vi "Power Meter Control Panel (No Objects).vi"(8 "error in (no error)":errorcluster) -> (0 "error out":errorcluster)   [LabVIEW 2012]
doc: "(Dynamic) A user-level application that simulates the physical front panel of the Instrument. Provide the user with buttons to manually control features of the instrument, and provide indicators of its current state."
uses:
  Newport 1830-C/Public/Filters.ctl
panel:
  in  "Which Filter":T1=1 items=["Orange"=1, "Green"=2, "Yellow"=3]
  out "Actual Power":dbl
  in  "Measured Power":dbl
  in  "Convert Power":bool
  in  "VISA Resource Name":refnum<visa-resource-name>="GPIB0::4::INSTR"
  out "Initialized?":bool
  in  "Filter":T1=1 items=["Orange"=1, "Green"=2, "Yellow"=3]
  out "Power":string
  in  "Time between Reads (ms)":i32=200
  in  "Read Continuous":bool
  in  "Averaging Time (s)":dbl=0.5
  in  "Averaging":bool
  out "Units":u16(ring)=1 items=["W"=1, "dB"=2, "dBm"=3, "REL"=4]
  out "AVG":u16(ring)=2 items=["Slow"=1, "Medium"=2, "Fast"=3]
  out "Run/Stop":u16(ring) items=["Stop", "Run"]
  out "ATTN":u16(ring) items=["Off", "On"]
  out "Local Lockout":u16(ring) items=["Off", "On"]
  out "Zero":u16(ring) items=["Off", "On"]
  out "Beeper":u16(ring) items=["Off", "On"]
  out "Backlight":u16(ring) items=["Off", "Low", "High"]
  out "Range":u16(ring) items=["Auto", "Highest Sensitivity", "30uW", "300uW", "3mW", "30mW", "300mW", "3W", "Lowest Sensitivity"]
  in  "Run/Stop set":u32(ring)=1 items=["Stop", "Run"]
  in  "ATTN set":u32(ring) items=["Off", "On"]
  in  "BKLT set":u32(ring)=1 items=["Off", "Low", "High"]
  in  "Range set":u32(ring) items=["Auto", "Highest Sensitivity", "30uW", "300uW", "3mW", "30mW", "300mW", "3W", "Lowest Sensitivity"]
  in  "Beeper set":u32(ring) items=["Off", "On"]
  in  "AVG set":u32(ring)=2 items=["Slow"=1, "Medium"=2, "Fast"=3]
  in  "Units set":u32(ring)=1 items=["W"=1, "dB"=2, "mdB"=3, "REL"=4]
  in  "Zero set":u32(ring) items=["Off", "On"]
  in  "Local set":u32(ring) items=["Off", "On"]
  in  "Read Current Power":bool
  in  "Set":bool
  in  "Read to \nControl":bool
  in  "Read":bool
  in  "Wavelength Set":dbl[unit]
  out "Wavelength":dbl[unit]
  in  "Copy actual to set":bool
  in  "Populate fields with member data":bool
  in  "stop":bool
  # "With \nAttn\nOn"
  # "Convert Measured Power"
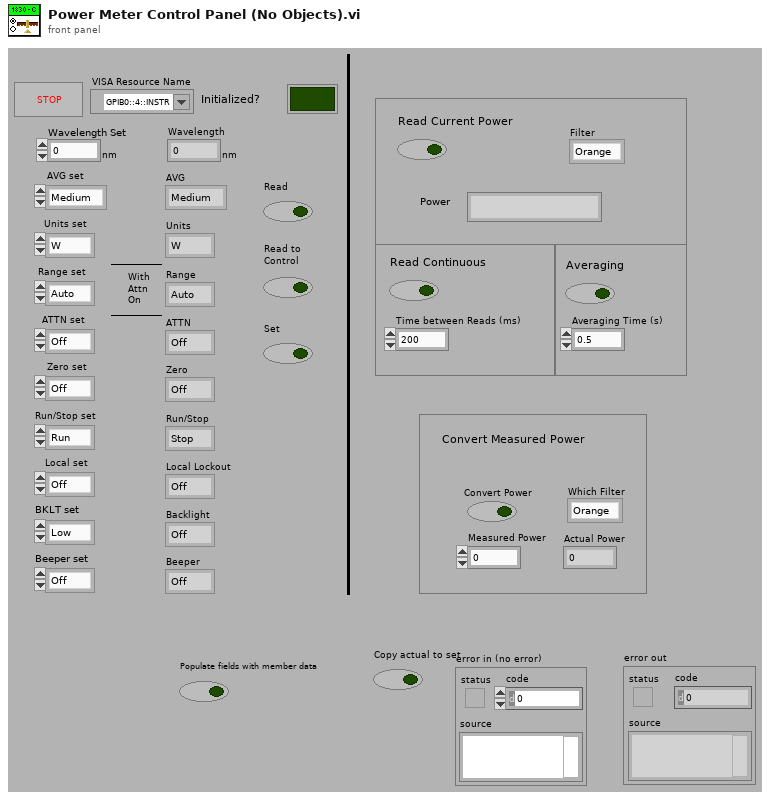
[diagram p1: front panel]
types:
  T1 = typedef "Filters.ctl" = u16
  T2 = cluster{"Wavelength":dbl[unit], "AVG":u16, "Range":u16, "Backlight":u16, "Beeper":u16, "Zero":u16, "Local Lockout":u16, "ATTN":u16, "Run/Stop":u16, "Units":u16, "Averaging Time":dbl, "Averaging":bool, "Most Recent Power":dbl, "Filter":T1}
  T3 = cluster{"Wavelength":dbl[unit], "AVG":i32, "Range":i32, "Backlight":i32, "Beeper":i32, "Zero":i32, "Local Lockout":i32, "ATTN":i32, "Run/Stop":i32, "Units":i32, "Averaging Time":dbl, "Averaging":bool, "Most Recent Power":dbl, "Filter":i32}
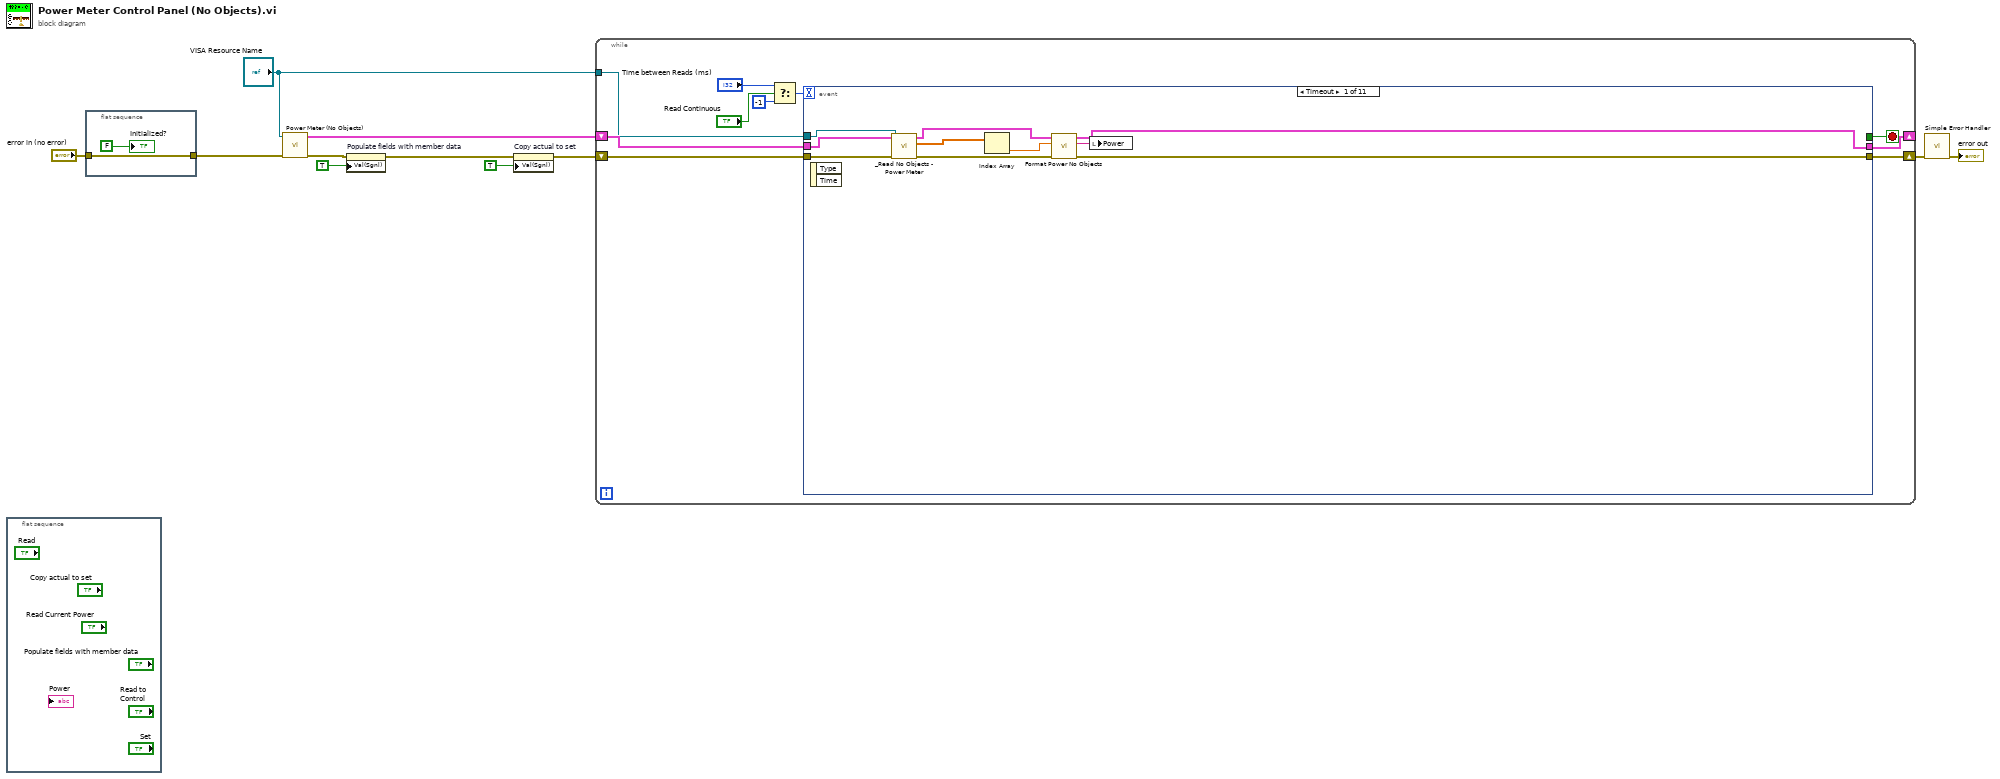
[diagram p0: block diagram]
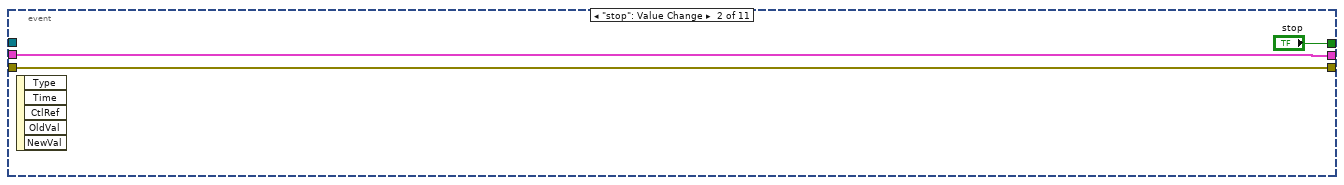
[diagram p2: hidden frame]
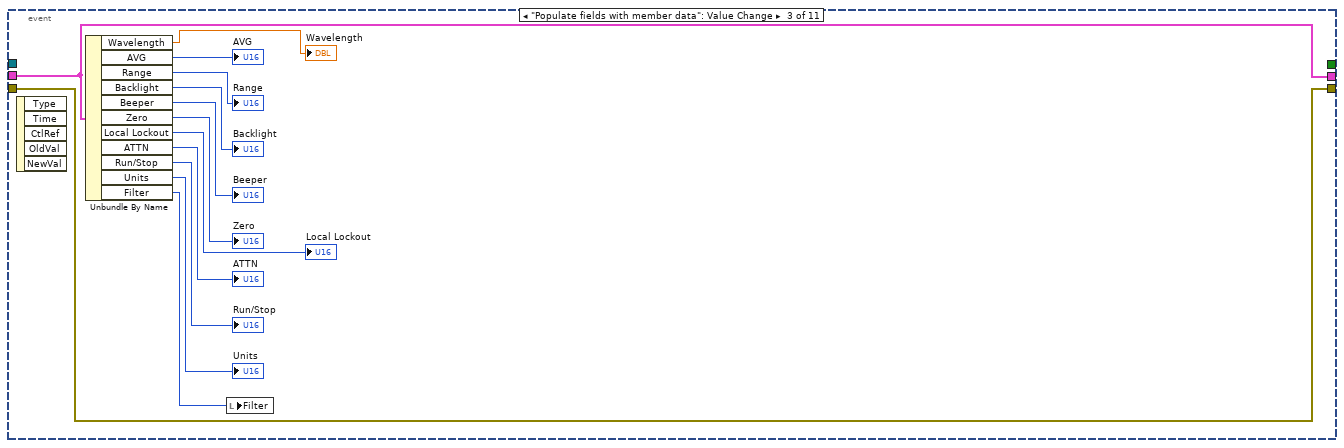
[diagram p3: hidden frame]
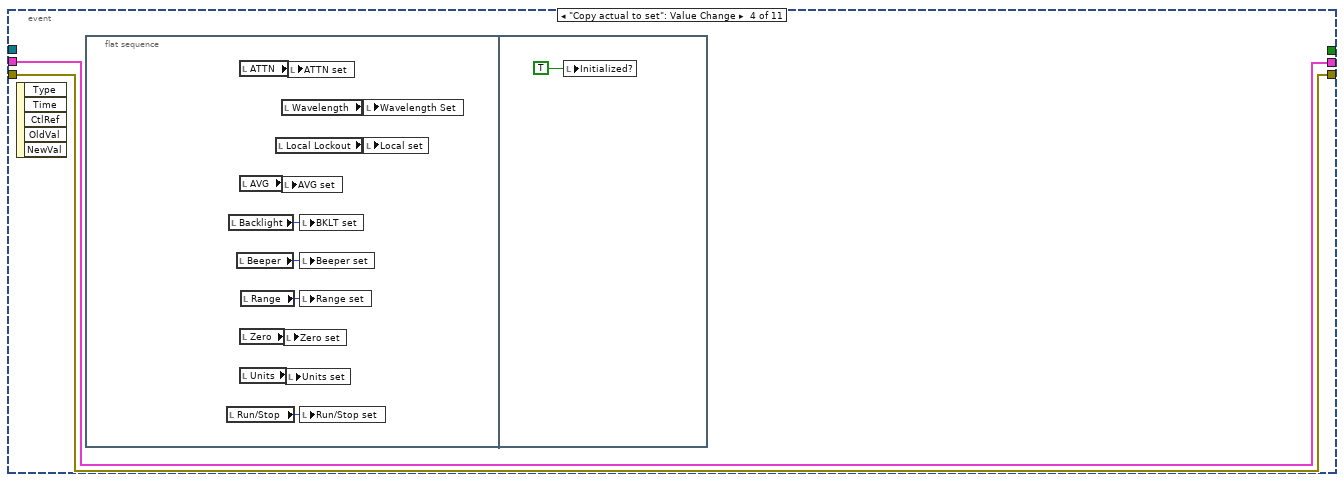
[diagram p4: hidden frame]
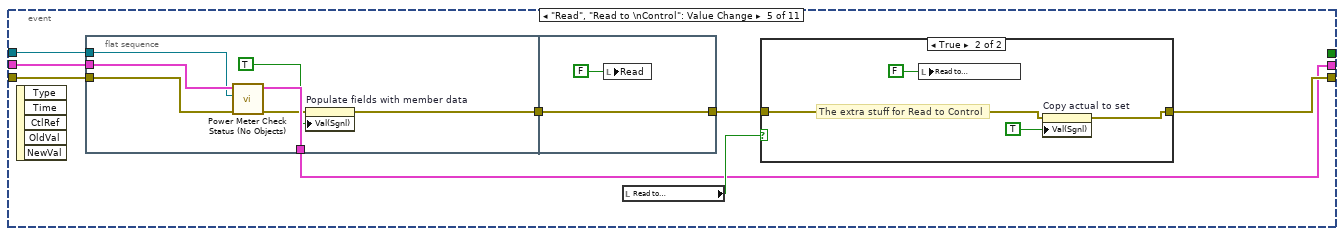
[diagram p5: hidden frame]
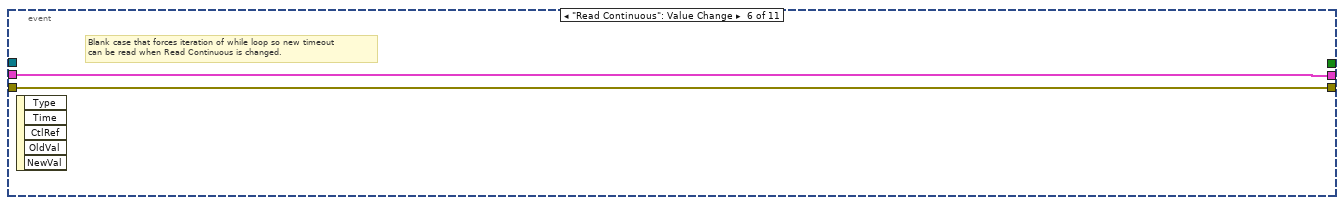
[diagram p7: hidden frame]
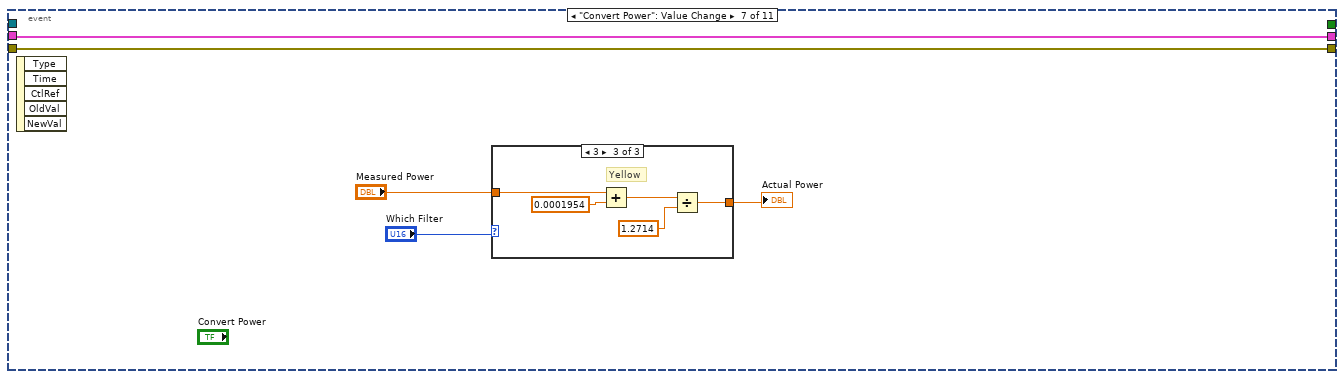
[diagram p8: hidden frame]
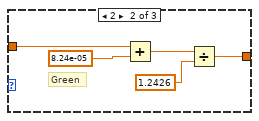
[diagram p10: hidden frame]
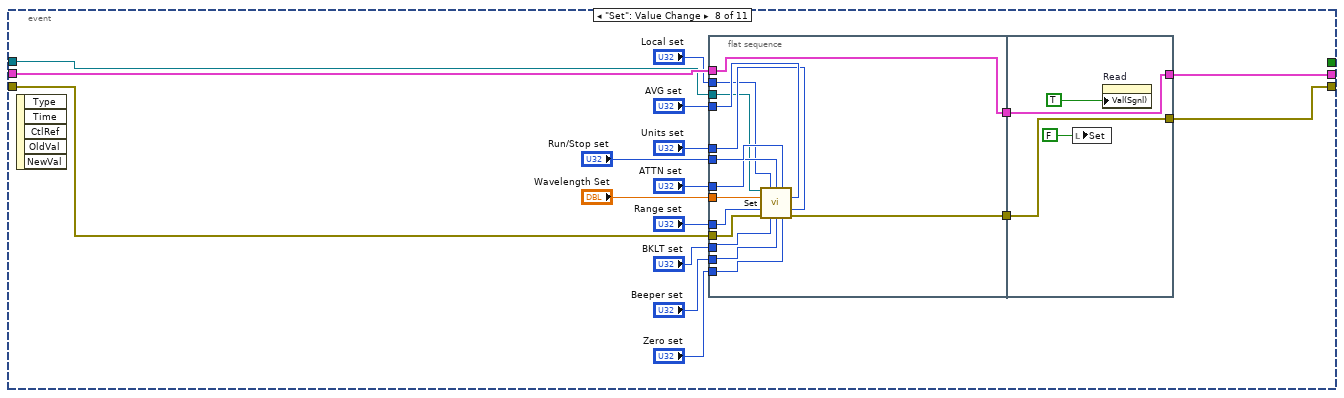
[diagram p11: hidden frame]
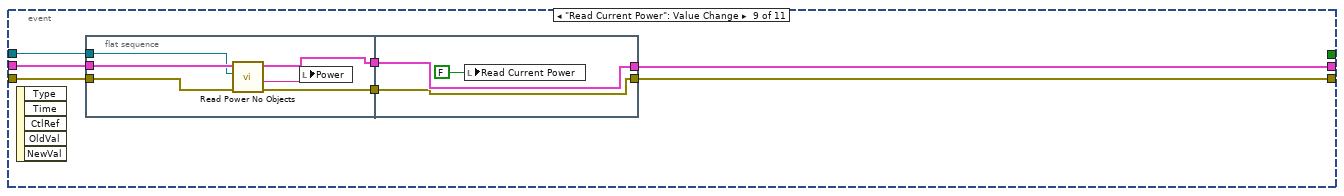
[diagram p12: hidden frame]
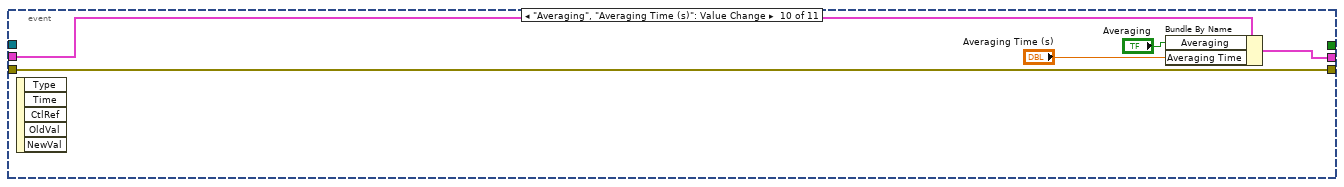
[diagram p13: hidden frame]
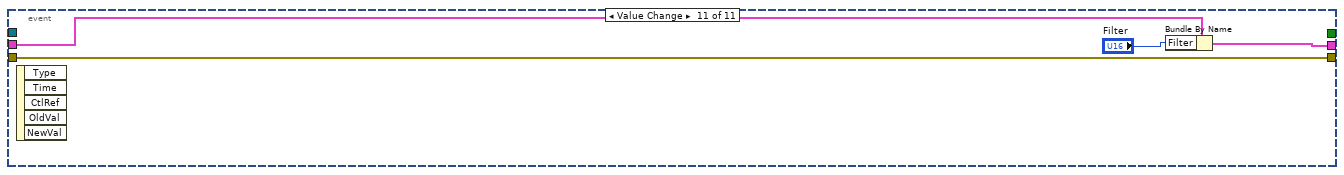
[diagram p14: hidden frame]
diagram:
  n1 = flat-sequence {
    frame #0 {
    }
  }
  n2 = flat-sequence {
    tunnel: "error in (no error)" -> [w12]
    tunnel: [w12] -> w4
    frame #0 {
      "Initialized?" <- FALSE
    }
  }
  n3 = call "Power Meter (No Objects).vi"("error in (no error)"=w4, "VISA resource name"="VISA Resource Name") -> ("error out"=w3:errorcluster, "Power Meter Out"=w2:T2)  [unwired: 8 in]
  n4 = property on="Populate fields with member data" class="Bool (strict)"(error in=w3, "Val(Sgnl)"=TRUE ("Value (Signaling)")) -> (error out=w9:errorcluster)  [unwired: 1 in, 1 out]
  n5 = property on="Copy actual to set" class="Bool (strict)"(error in=w9, "Val(Sgnl)"=TRUE ("Value (Signaling)")) -> (error out=w8:errorcluster)  [unwired: 1 in, 1 out]
  n6 = while {
    shift-right: [w20] -> _
    shift-left: w2 -> [w22]
    shift-right: [w19] -> w7
    shift-left: w8 -> [w21]
    tunnel: "VISA Resource Name" -> [w14]
    stop <- w23 stop-if-true
    n7 = Select(t="Time between Reads (ms)", s="Read Continuous", f=-1) -> (s? t:f=w16:i32)
    n8 = event shown="[0] Timeout" {
      selector: _ -> [_ _ _ _ _ _ _ _ _ _ _]
      dyn-events: _ -> [_ _ _ _ _ _ _ _ _ _ _]
      timeout: w16 -> [_ _ _ _ _ _ _ _ _ _ _]
      tunnel: [_ "stop" _ _ _ _ _ _ _ _ _] -> w23
      tunnel: [w27 w35 w48 w51 w64 w86 w90 w116 w140 w157 w159] -> w20
      tunnel: w22 -> [w25 w35 w48 w51 w70 w86 w90 w119 w144 w158 w162]
      tunnel: [w28 w34 w47 w50 w65 w85 w91 w115 w139 w156 w160] -> w19
      tunnel: w21 -> [w33 w34 w47 w50 w69 w85 w91 w117 w142 w156 w160]
      tunnel: w14 -> [w26 _ _ _ w63 _ _ w104 w138 _ _]
      event Timeout {
        n9 = event-data() -> ()  [unwired: 1 in, 2 out]
        n10 = call "_Read No Objects - Power Meter.vi"("error in (no error)"=w33, "VISA Resource Name In"=w26, "Power Meter in"=w25) -> ("error out"=w32:errorcluster, "X array"=w31:dbl[], "Power Meter Out"=w24:T3)  [unwired: 6 in]
        n11 = Index Array(array=w31) -> (element=w30:dbl)  [unwired: 1 in]
        n12 = call "Format Power No Objects.vi"("error in"=w32, "Power"=w30, "Cluster In"=w24) -> ("error out"=w28:errorcluster, "Formatted Power"=w29:string, "Cluster Out"=w27:T2)  [unwired: 6 in]
        n13 = local write "Power"(w29) -> ()
      }
      event "stop": Value Change {
        n14 = event-data() -> ()  [unwired: 1 in, 5 out]
      }
      event "Populate fields with member data": Value Change {
        n15 = event-data() -> ()  [unwired: 1 in, 5 out]
        n16 = Unbundle By Name(w48) -> ("Wavelength"=→"Wavelength":dbl[unit], "AVG"=→"AVG":u16, "Range"=→"Range":u16, "Backlight"=→"Backlight":u16, "Beeper"=→"Beeper":u16, "Zero"=→"Zero":u16, "Local Lockout"=→"Local Lockout":u16, "ATTN"=→"ATTN":u16, "Run/Stop"=→"Run/Stop":u16, "Units"=→"Units":u16, "Filter"=w37:T1)
        n17 = local write "Filter"(w37) -> ()
      }
      event "Copy actual to set": Value Change {
        n18 = event-data() -> ()  [unwired: 1 in, 5 out]
        n19 = flat-sequence {
          frame #0 {
            n20 = local read "Run/Stop"() -> (w55:u16)
            n21 = local read "Backlight"() -> (w59:u16)
            n22 = local read "Beeper"() -> (w58:u16)
            n23 = local read "ATTN"() -> (w53:u16)
            n24 = local read "AVG"() -> (w60:u16)
            n25 = local read "Zero"() -> (w52:u16)
            n26 = local read "Units"() -> (w54:u16)
            n27 = local read "Range"() -> (w56:u16)
            n28 = local read "Local Lockout"() -> (w57:u16)
            n29 = local read "Wavelength"() -> (w61:dbl[unit])
            n30 = local write "AVG set"(w60) -> ()
            n31 = local write "Zero set"(w52) -> ()
            n32 = local write "Units set"(w54) -> ()
            n33 = local write "ATTN set"(w53) -> ()
            n34 = local write "BKLT set"(w59) -> ()
            n35 = local write "Beeper set"(w58) -> ()
            n36 = local write "Range set"(w56) -> ()
            n37 = local write "Run/Stop set"(w55) -> ()
            n38 = local write "Wavelength Set"(w61) -> ()
            n39 = local write "Local set"(w57) -> ()
          }
          frame #1 {
            n40 = local write "Initialized?"(TRUE ("Power\nMeter\nInitialized?")) -> ()
          }
        }
      }
      event "Read", "Read to \nControl": Value Change {
        n41 = event-data() -> ()  [unwired: 1 in, 5 out]
        n42 = flat-sequence {
          tunnel: w70 -> [w82]
          tunnel: w69 -> [w81]
          tunnel: [w78] -> w66
          tunnel: [w80] -> w64
          tunnel: w63 -> [w76]
          tunnel: [w83] -> w67
          tunnel: w66 -> [w83]
          frame #0 {
            n43 = call "Power Meter Check Status (No Objects).vi"("error in (no error)"=w81, "VISA resource name"=w76, "Cluster In"=w82) -> ("error out"=w79:errorcluster, "Cluster Out"=w80:T2)  [unwired: 6 in, 1 out]
            n44 = property on="Populate fields with member data" class="Bool (strict)"(error in=w79, "Val(Sgnl)"=TRUE ("Value (Signaling)")) -> (error out=w78:errorcluster)  [unwired: 1 in, 1 out]
          }
          frame #1 {
            n45 = local write "Read"(FALSE ("Read")) -> ()
          }
        }
        n46 = local read "Read to \nControl"() -> (w68:bool)
        n47 = case shown="True" w68 {
          tunnel: w67 -> [w71 w73]
          tunnel: [w71 w72] -> w65
          frame False {
          }
          frame True {
            # "The extra stuff for Read to Control"
            n48 = local write "Read to \nControl"(FALSE ("Read")) -> ()
            n49 = property on="Copy actual to set" class="Bool (strict)"(error in=w73, "Val(Sgnl)"=TRUE ("Value (Signaling)")) -> (error out=w72:errorcluster)  [unwired: 1 in, 1 out]
          }
        }
      }
      event "Read Continuous": Value Change {
        # "Blank case that forces iteration of while loop so new timeout\ncan be read when Read Continuous is changed."
        n50 = event-data() -> ()  [unwired: 1 in, 5 out]
      }
      event "Convert Power": Value Change {
        n51 = event-data() -> ()  [unwired: 1 in, 5 out]
        n52 = case shown="3" "Which Filter" {
          tunnel: "Measured Power" -> [w92 w94 w99]
          tunnel: [w92 w93 w98] -> w88
          frame 1, Default {
            # "Orange"
          }
          frame 2 {
            # "Green"
            n53 = Add(x=w94, y=8.24e-05) -> (x+y=w95:dbl)
            n54 = Divide(x=w95, y=1.2426) -> (x/y=w93:dbl)
          }
          frame 3 {
            # "Yellow"
            n55 = Add(x=w99, y=0.0001954) -> (x+y=w100:dbl)
            n56 = Divide(x=w100, y=1.2714) -> (x/y=w98:dbl)
          }
        }
        "Actual Power" <- w88
      }
      event "Set": Value Change {
        n57 = event-data() -> ()  [unwired: 1 in, 5 out]
        n58 = flat-sequence {
          tunnel: w119 -> [w122]
          tunnel: [w121] -> w118
          tunnel: w117 -> [w120]
          tunnel: "AVG set" -> [w133]
          tunnel: "Units set" -> [w132]
          tunnel: "Run/Stop set" -> [w131]
          tunnel: "ATTN set" -> [w130]
          tunnel: "Local set" -> [w129]
          tunnel: "Wavelength Set" -> [w128]
          tunnel: "Range set" -> [w127]
          tunnel: "BKLT set" -> [w126]
          tunnel: "Beeper set" -> [w125]
          tunnel: "Zero set" -> [w124]
          tunnel: w104 -> [w123]
          tunnel: [w122] -> w103
          tunnel: [w134] -> w116
          tunnel: [w135] -> w115
          tunnel: w118 -> [w135]
          tunnel: w103 -> [w134]
          frame #0 {
            n59 = call "Set.vi"("VISA resource name"=w123, "Local Lockout (0:1)"=w129, "ATTN (0:1)"=w130, "Run/Stop (1:0)"=w131, "Wavelength (nnnn)"=w128, "AVG (1:3)"=w133, "Range (0-Auto,1:8)"=w127, "Units (1:4)"=w132, "error in (no error)"=w120, "Backlight (0:2)"=w126, "Beeper (0:1)"=w125, "Zero (0:1)"=w124) -> ("error out"=w121:errorcluster)  [unwired: 2 in, 1 out]
          }
          frame #1 {
            n60 = local write "Set"(FALSE ("Set")) -> ()
            n61 = property on="Read" class="Bool (strict)"("Val(Sgnl)"=TRUE ("Value (Signaling)")) -> ()  [unwired: 2 in, 2 out]
          }
        }
      }
      event "Read Current Power": Value Change {
        n62 = event-data() -> ()  [unwired: 1 in, 5 out]
        n63 = flat-sequence {
          tunnel: w144 -> [w146]
          tunnel: [w147] -> w143
          tunnel: w142 -> [w150]
          tunnel: [w148] -> w141
          tunnel: w138 -> [w145]
          tunnel: [w152] -> w140
          tunnel: w143 -> [w152]
          tunnel: [w151] -> w139
          tunnel: w141 -> [w151]
          frame #0 {
            n64 = call "Read Power No Objects.vi"("error in (no error)"=w150, "VISA Resource Name"=w145, "Cluster In"=w146) -> ("error out"=w148:errorcluster, "Current Power w/ Units"=w149:string, "Cluster Out"=w147:T2)  [unwired: 5 in, 1 out]
            n65 = local write "Power"(w149) -> ()
          }
          frame #1 {
            n66 = local write "Read Current Power"(FALSE ("Read Current Value")) -> ()
          }
        }
      }
      event "Averaging", "Averaging Time (s)": Value Change {
        n67 = event-data() -> ()  [unwired: 1 in, 5 out]
        n68 = Bundle By Name(cluster=w158, "Averaging"="Averaging", "Averaging Time"="Averaging Time (s)") -> (w157:T2)
      }
      event Value Change {
        n69 = event-data() -> ()  [unwired: 1 in, 5 out]
        n70 = Bundle By Name(cluster=w162, "Filter"="Filter") -> (w159:T2)
      }
    }
  }
  n71 = call <vilib>:"Simple Error Handler.vi"("error in (no error)"=w7) -> ("error out"=→"error out":errorcluster)  [unwired: 1 in, 7 out]
